vi "Container_init.vi"(1 "Container Properties":T1[](array[typedef])=[{"#C_ID"=0.0, "Dimensions"=[10.0, 10.0], "Space"=[]}, {"#C_ID"=0.0, "Dimensions"=[20.0, 20.0], "Space"=[]}]) -> (0 "Array":T1[](array[typedef])=[{"#C_ID"=0.0, "Dimensions"=[10.0, 10.0], "Space"=[[FALSE, FALSE, FALSE, FALSE, FALSE, FALSE, FALSE, FALSE, FALSE, FALSE], [FALSE, FALSE, FALSE, FALSE, FALSE, FALSE, FALSE, FALSE, FALSE, FALSE]]}, {"#C_ID"=0.0, "Dimensions"=[20.0, 20.0], "Space"=[[FALSE, FALSE, FALSE, FALSE, FALSE, FALSE, FALSE, FALSE, FALSE, FALSE, FALSE, FALSE, FALSE, FALSE, FALSE, FALSE, FALSE, FALSE, FALSE, FALSE], [FALSE, FALSE, FALSE, FALSE, FALSE, FALSE, FALSE, FALSE, FALSE, FALSE, FALSE, FALSE, FALSE, FALSE, FALSE, FALSE, FALSE, FALSE, FALSE, FALSE]]}])   [LabVIEW 2015]
uses:
  Controls/Container_Properties.ctl
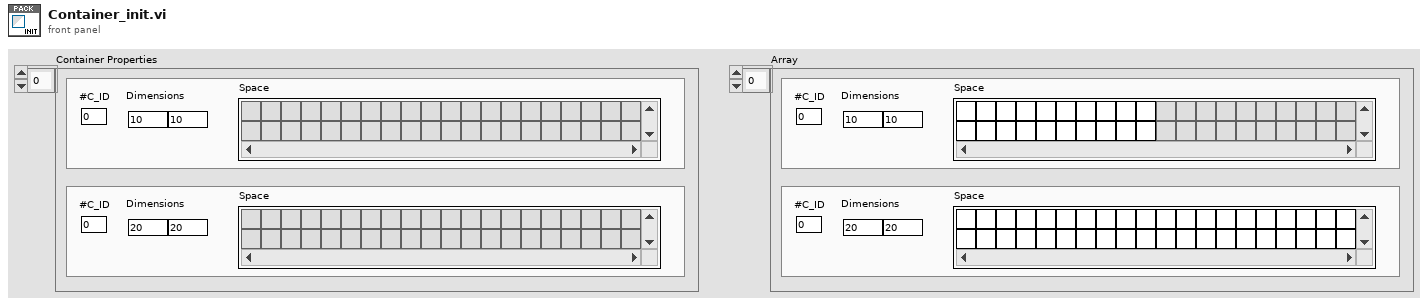
[diagram p1: front panel]
types:
  T1 = typedef "Container_Properties.ctl" = cluster{"#C_ID":dbl, "Dimensions":dbl[], "Space":bool[][]}
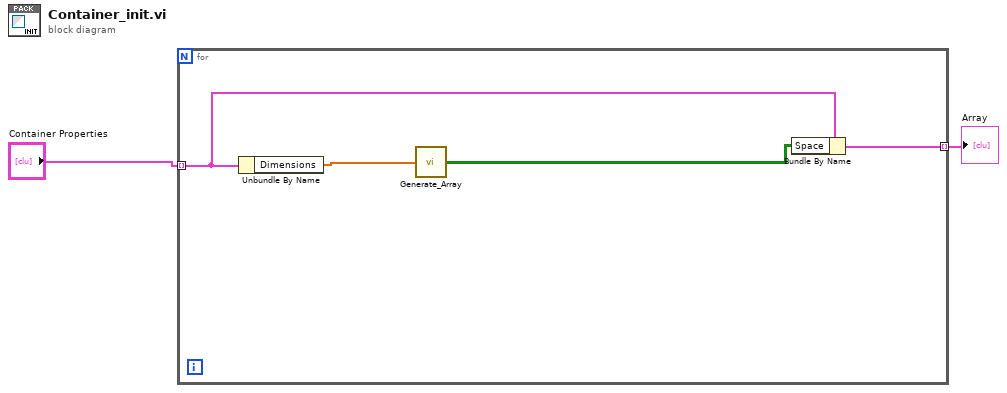
[diagram p0: block diagram]
diagram:
  n1 = for {
    tunnel: "Container Properties" -> [w6] mode=indexing
    tunnel: [w5] -> w2 mode=indexing
    n2 = Unbundle By Name(w6) -> ("Dimensions"=w4:dbl[])
    n3 = call "Generate_Array.vi"("Dimensions"=w4) -> ("Array"=w3:bool[][])
    n4 = Bundle By Name(cluster=w6, "Space"=w3) -> (w5:T1)
  }
  "Array" <- w2
